vi "RSZVB Rename Calibration Kit.vi"(7 "New Label (\"\")":string, 8 "error in (no error)":errorcluster {"code" format="%.0x"}, 9 "Label (\"\")":string, 10 "Calibration Kit Name (\"\")":string, 11 "VISA session":refnum<visa-resource-name>) -> (0 "error out":errorcluster {"code" format="%.0x"}, 3 "dup VISA session":refnum<visa-resource-name>)   [LabVIEW 2011]
doc: "This VI renames an existing calibration kit label. \n\nRemote-control command(s):\n[SENSe<Ch>:]CORRection:CKIT:LLABel"
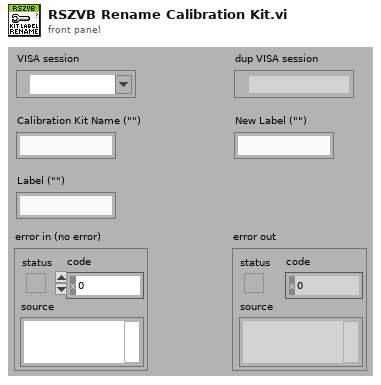
[diagram p1: front panel]
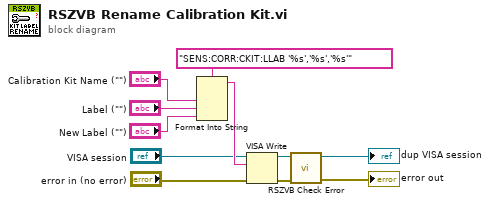
[diagram p0: block diagram]
diagram:
  n1 = Format Into String(format string="SENS:CORR:CKIT:LLAB '%s','%s','%s'", "Calibration Kit Name (\"\")", "Label (\"\")", "New Label (\"\")") -> (resulting string=w11:string)  [unwired: 2 in, 1 out]
  n2 = VISA Write(VISA resource name="VISA session", write buffer=w11, error in (no error)="error in (no error)") -> (VISA resource name out=w9:refnum<visa-resource-name>, error out=w10:errorcluster)  [unwired: 1 out]
  n3 = call "RSZVB Check Error.vi"("error in (no error)"=w10, "VISA session"=w9) -> ("error out"=→"error out":errorcluster, "dup VISA session"=→"dup VISA session":refnum<visa-resource-name>)  [unwired: 8 in]
